vi "S1500_S7Com_TriggerUngerade.vi"(8 "error in (no error)":errorcluster caption="Fehler (Eingang, kein Fehler)", 11 "INT":i32) -> (0 "error out":errorcluster caption="Fehler (Ausgang)", 3 "Boolesch":bool)   [LabVIEW 2018]
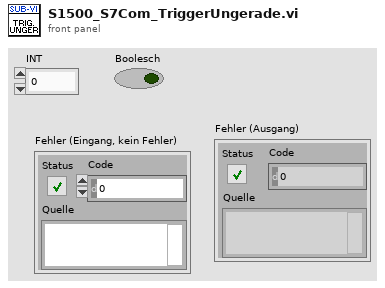
[diagram p1: front panel]
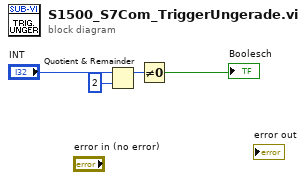
[diagram p0: block diagram]
diagram:
  n1 = Quotient & Remainder(x="INT", y=2) -> (x-y*floor(x/y)=w2:i32)  [unwired: 1 out]
  n2 = Not Equal To 0?(x=w2) -> (x != 0?=→"Boolesch":bool)
